vi "Pre-Dig.vi"(6 "Search Path":path[](array[path]), 8 "Error In":errorcluster, 10 "Selection List[] In":refnum<vi>[](array[refnum]), 11 "VI In":refnum<vi>) -> (0 "Error Out":errorcluster, 2 "Selection List[] Out":refnum<vi>[](array[refnum]), 3 "VI Out":refnum<vi>)   [LabVIEW 2018, in "Toolkit.lvlib"]
uses:
  Toolkit.lvlib
  Typedefs/Hooks.ctl
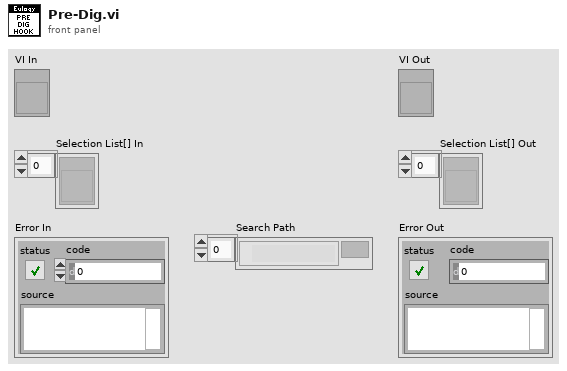
[diagram p1: front panel]
types:
  T1 = typedef "Toolkit.lvlib/Hooks.ctl" = enum16{"Pre-Dig", "Post-Dig", "Pre-Reanimate", "Post-Reanimate", "Pre-Smite", "Post-Smite", "Pre-Bury", "Post-Bury"}
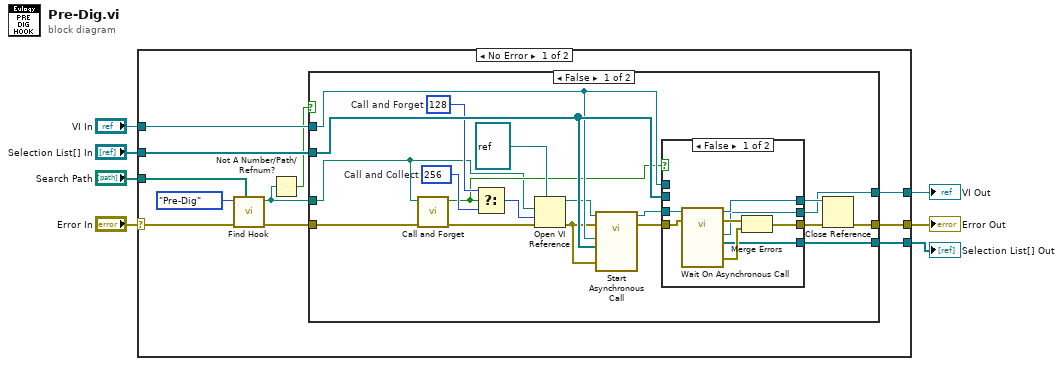
[diagram p0: block diagram]
diagram:
  n1 = case shown="No Error" "Error In" {
    selector: "Error In" -> [w16 w55]
    tunnel: [w17 w55] -> w7
    tunnel: "VI In" -> [w12 w54]
    tunnel: "Selection List[] In" -> [w13 w53]
    tunnel: [w15 w53] -> w3
    tunnel: [w14 w54] -> w2
    tunnel: "Search Path" -> [w10 _]
    frame No Error {
      n2 = call "Find Hook.vi"("Search Path"=w10, "Error In"=w16, "Hook"=Hooks."Pre-Dig") -> ("Error Out"=w18:errorcluster, "Hook"=w9:path)  [unwired: 7 in]
      n3 = Not A Number/Path/Refnum?(number/path/refnum=w9) -> (NaN/Path/Refnum?=w8:bool)
      n4 = case shown="False" w8 {
        tunnel: w9 -> [w19 _]
        tunnel: w18 -> [w24 w51]
        tunnel: [w36 w51] -> w17
        tunnel: [w31 w50] -> w15
        tunnel: [w30 w52] -> w14
        tunnel: w13 -> [w29 w50]
        tunnel: w12 -> [w28 w52]
        frame False {
          w26 = 256  # Call and Collect
          w27 = 128  # Call and Forget
          n5 = call "Call and Forget.vi"("Error In"=w24, "Hook"=w19) -> ("Error Out"=w23:errorcluster, "Call and Forget"=w22:bool)  [unwired: 8 in]
          n6 = Select(t=w27, s=w22, f=w26) -> (s? t:f=w25:i32)
          n7 = Open VI Reference(type specifier VI Refnum (for type only)=refnum<vi> refnum, vi path=w19, options=w25, error in (no error)=w23) -> (vi reference=w21:refnum<vi>, error out=w20:errorcluster)  [unwired: 2 in]
          n8 = call-by-ref "Start Asynchronous Call"(reference=w21, error in=w20, "Error In"=w20, "Selection List[] In"=w29, "VI In"=w28) -> (reference out=w35:refnum<vi>, error out=w33:errorcluster)  [unwired: 6 in, 3 out]
          n9 = case shown="False" w22 {
            tunnel: w35 -> [w45 w49]
            tunnel: [w44 w49] -> w34
            tunnel: w33 -> [w43 w48]
            tunnel: [w41 w48] -> w32
            tunnel: [w39 w47] -> w31
            tunnel: [w38 w46] -> w30
            tunnel: w29 -> [_ w47]
            tunnel: w28 -> [_ w46]
            frame False {
              n10 = call-by-ref "Wait On Asynchronous Call"(reference=w45, error in=w43) -> (reference out=w44:refnum<vi>, error out=w42:errorcluster, "Error Out"=w40:errorcluster, "Selection List[] Out"=w39:refnum<vi>[], "VI Out"=w38:refnum<vi>)  [unwired: 9 in]
              n11 = Merge Errors(w42, w40) -> (w41:errorcluster)
            }
            frame True {
            }
          }
          n12 = Close Reference(reference=w34, error in (no error)=w32) -> (error out=w36:errorcluster)
        }
        frame True {
        }
      }
    }
    frame Error {
    }
  }
  "Error Out" <- w7
  "Selection List[] Out" <- w3
  "VI Out" <- w2
